vi "Read Spectrum and Save It_backup.vi"(0 "VISA Session":refnum<visa-resource-name>, 6 "Pasta Destino DESTA aquisicao":path=path "d:/Users/Stinky/Documents", 9 "Corrente Atual (mA)":dbl, 11 "Error In":errorcluster, 12 "Iteracao":i32) -> (4 "Copy VISA Session":refnum<visa-resource-name>, 8 "PxI":dbl[](array[numeric]), 10 "XY Graph":T1(graph), 15 "Error Out":errorcluster)   [LabVIEW 2018]
panel:
  out "Return Data Bytes 2":u16
  out "Wavelike Data (X)":dbl[](array[numeric]) format="%.12f"
  out "Return All Data 2":string
  out "Wavelike Data (Y)":dbl[](array[numeric]) format="%.12f"
  out "Return Data Bytes":u16
  out "Return All Data":string
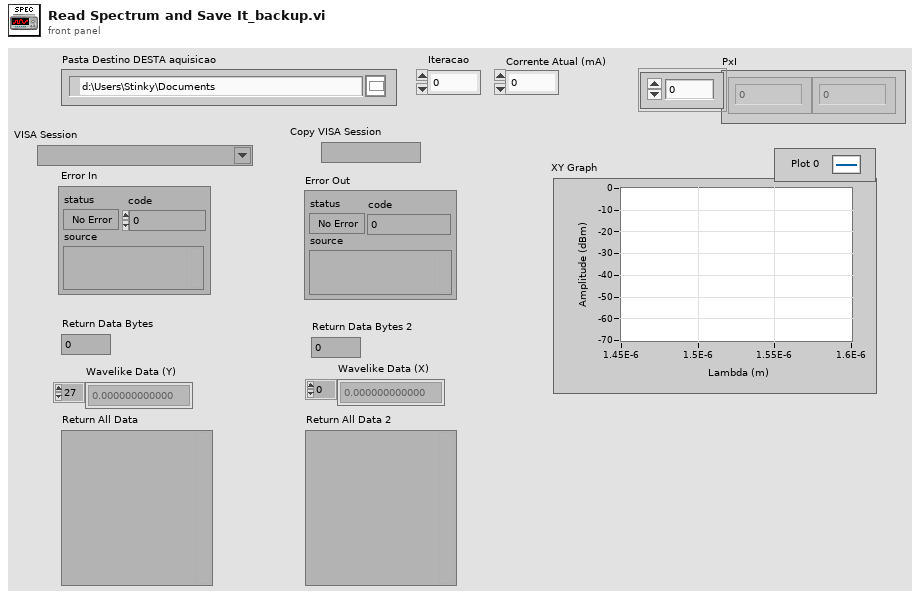
[diagram p1: front panel]
types:
  T1 = cluster{"Wavelike Data":dbl[], "Wavelike Data":dbl[]}
  T2 = enum16{"Y AXIS Data Output", "X AXIS Data Output"}
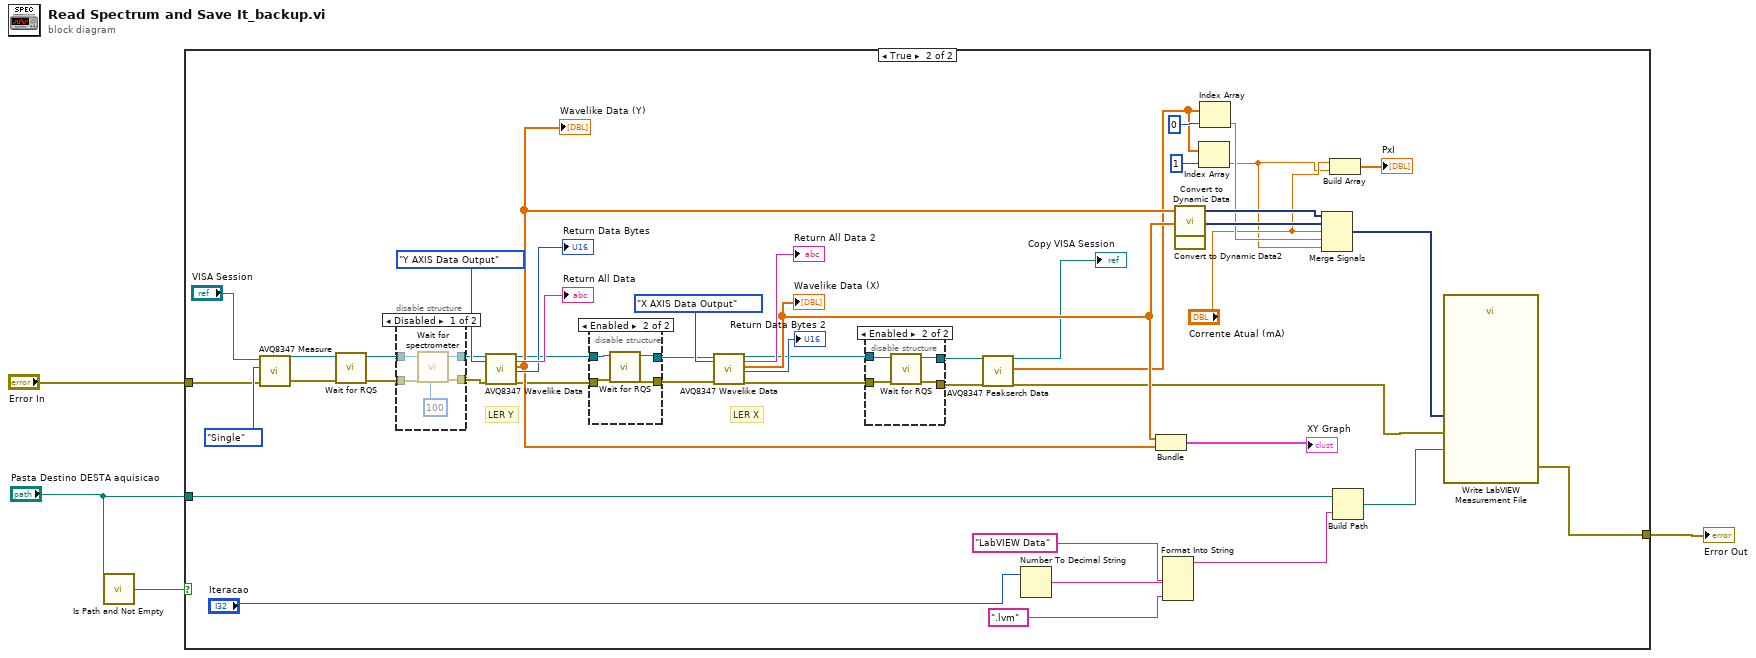
[diagram p0: block diagram]
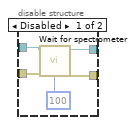
[diagram p3: hidden frame]
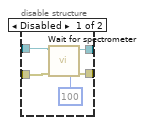
[diagram p4: hidden frame]
diagram:
  n1 = call <vilib>:"Is Path and Not Empty.vi"("path"="Pasta Destino DESTA aquisicao") -> ("Is Path and Not Empty?"=w3:bool)  [unwired: 4 in]
  n2 = case shown="True" w3 {
    tunnel: "Pasta Destino DESTA aquisicao" -> [_ w42]
    tunnel: "Error In" -> [w5 w28]
    tunnel: [w5 w27] -> w1
    frame False {
    }
    frame True {
      # "LER X"
      # "LER Y"
      n3 = call "AVQ8347 Measure.vi"("Error In"=w28, "Measure Select"=enum16{"Stop", "Single", "Repeat"}."Single", "VISA Session"="VISA Session") -> ("Error Out"=w8:errorcluster, "Copy VISA Session"=w9:refnum<visa-resource-name>)  [unwired: 6 in, 1 out]
      n4 = call <vilib>:"Wait for RQS.vi"("error in (no error)"=w8, "VISA resource name"=w9) -> ("error out"=w7:errorcluster, "VISA resource name out"=w6:refnum<visa-resource-name>)  [unwired: 7 in, 1 out]
      n5 = disable-structure shown="Disabled" {
        disable-tunnel: [w74 w76] -> w34
        disable-tunnel: [w73 w75] -> w33
        disable-tunnel: w7 -> [w71 w75]
        disable-tunnel: w6 -> [w70 w76]
        frame Disabled {
          n6 = call "Wait for spectrometer.vi"("error in (no error)"=w71, "milliseconds to wait"=u32 100, "VISA Refnum in"=w70) -> ("error out"=w73:errorcluster, "VISA Refnum out"=w74:refnum<visa-resource-name>)  [unwired: 6 in, 1 out]
        }
        frame Enabled {
        }
      }
      n7 = call "AVQ8347 Wavelike Data.vi"("VISA Session"=w34, "Axis Select"=T2."Y AXIS Data Output", "Error In"=w33) -> ("Copy VISA Session"=w13:refnum<visa-resource-name>, "Return All Data"=→"Return All Data":string, "Wavelike Data"=w40:dbl[], "Return Data Bytes"=→"Return Data Bytes":u16, "Error Out"=w29:errorcluster)  [unwired: 12 in]
      "Wavelike Data (Y)" <- w40
      n8 = disable-structure shown="Enabled" {
        disable-tunnel: [w64 w66] -> w31
        disable-tunnel: [w63 w67] -> w30
        disable-tunnel: w29 -> [w62 w68]
        disable-tunnel: w13 -> [w61 w69]
        frame Disabled {
          n9 = call "Wait for spectrometer.vi"("error in (no error)"=w62, "milliseconds to wait"=u32 100, "VISA Refnum in"=w61) -> ("error out"=w63:errorcluster, "VISA Refnum out"=w64:refnum<visa-resource-name>)  [unwired: 6 in, 1 out]
        }
        frame Enabled {
          n10 = call <vilib>:"Wait for RQS.vi"("error in (no error)"=w68, "VISA resource name"=w69) -> ("error out"=w67:errorcluster, "VISA resource name out"=w66:refnum<visa-resource-name>)  [unwired: 7 in, 1 out]
        }
      }
      n11 = call "AVQ8347 Wavelike Data.vi"("VISA Session"=w31, "Axis Select"=T2."X AXIS Data Output", "Error In"=w30) -> ("Copy VISA Session"=w12:refnum<visa-resource-name>, "Return All Data"=→"Return All Data 2":string, "Wavelike Data"=w41:dbl[], "Return Data Bytes"=→"Return Data Bytes 2":u16, "Error Out"=w26:errorcluster)  [unwired: 12 in]
      "Wavelike Data (X)" <- w41
      n12 = disable-structure shown="Enabled" {
        disable-tunnel: w26 -> [w55 w59]
        disable-tunnel: [w54 w57] -> w24
        disable-tunnel: [w53 w58] -> w23
        disable-tunnel: w12 -> [w52 w60]
        frame Disabled {
          n13 = call "Wait for spectrometer.vi"("error in (no error)"=w55, "milliseconds to wait"=u32 100, "VISA Refnum in"=w52) -> ("error out"=w53:errorcluster, "VISA Refnum out"=w54:refnum<visa-resource-name>)  [unwired: 6 in, 1 out]
        }
        frame Enabled {
          n14 = call <vilib>:"Wait for RQS.vi"("error in (no error)"=w59, "VISA resource name"=w60) -> ("error out"=w58:errorcluster, "VISA resource name out"=w57:refnum<visa-resource-name>)  [unwired: 7 in, 1 out]
        }
      }
      n15 = call "AVQ8347 Peakserch Data.vi"("VISA Session"=w24, "Error In"=w23) -> ("Copy VISA Session"=→"Copy VISA Session":refnum<visa-resource-name>, "Peakserch Data"=w17:dbl[], "Error Out"=w22:errorcluster)  [unwired: 13 in, 2 out]
      n16 = Number To Decimal String(number="Iteracao") -> (decimal integer string=w11:string)  [unwired: 1 in]
      n17 = Bundle("Wavelike Data"=w41, "Wavelike Data"=w40) -> (→"XY Graph":T1)  [unwired: 1 in]
      n18 = Format Into String("LabVIEW Data", w11, ".lvm") -> (resulting string=w36:string)  [unwired: 3 in, 1 out]
      n19 = call "Convert to Dynamic Data"("Array"=w40) -> ("Dynamic Data Type"=w44:dynamicdata)  [unwired: 3 in]
      n20 = call "Convert to Dynamic Data2"("Array"=w41) -> ("Dynamic Data Type"=w43:dynamicdata)  [unwired: 3 in]
      n21 = Index Array(array=w17, index=1) -> (element=w15:dbl)
      n22 = Index Array(array=w17, index=0) -> (element=w19:dbl)
      n23 = Merge Signals(w44, w43, "Corrente Atual (mA)", w19, w15) -> (w45:dynamicdata)
      n24 = Build Array("Corrente Atual (mA)", w15) -> (→"PxI":dbl[])
      n25 = Build Path(base path=w42, name or relative path=w36) -> (appended path=w25:path)
      n26 = call "Write LabVIEW Measurement File"("Signals"=w45, "error in (no error)"=w22, "Filename"=w25) -> ("error out"=w27:errorcluster)  [unwired: 14 in, 2 out]
    }
  }
  "Error Out" <- w1
